vi "Read shortStatus.vi"(8 "error in (no error)":errorcluster, 11 "DomeController in":refnum<class "DomeController.lvclass">) -> (0 "error out":errorcluster, 2 "shortStatus":T1 {"azimuthAngle" min=0.0 max=360.0; "openingPercentage" min=0.0 max=100.0; "mainDoorOpeningPercentage" min=0.0 max=100.0}, 3 "DomeController out":refnum<class "DomeController.lvclass">)   [LabVIEW 2016, in "DomeController.lvclass"]
uses:
  DomeController.lvclass
  domeCommunicator/ComTypedefs/shortStatus.ctl
  domeCommunicator/ComTypedefs/openingStates.ctl
  IDome/domeTypedefs/openingPercentage.ctl
  domeCommunicator/ComTypedefs/sensorCode.ctl
  domeCommunicator/ComTypedefs/azimimuthPositionStatus.ctl
  IDome/domeTypedefs/azimuth.ctl
  IDome/domeTypedefs/direction.ctl
  IDome/domeTypedefs/domeState.ctl
  IDome/domeTypedefs/motionDirection.ctl
  IDome/domeTypedefs/openingMotion.ctl
  DomeController.lvclass/DomeController.ctl
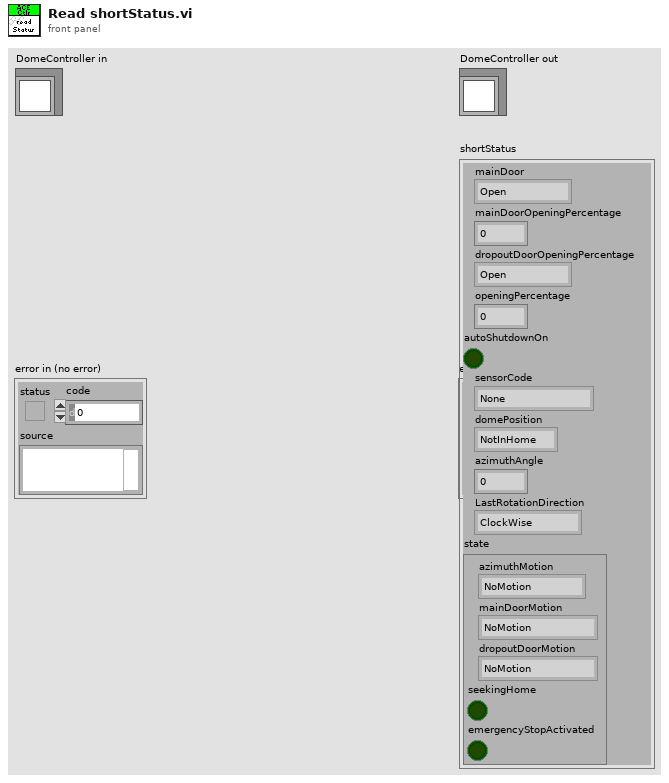
[diagram p1: front panel]
types:
  T1 = typedef "shortStatus.ctl" = cluster{"mainDoor":T2, "mainDoorOpeningPercentage":T3, "dropoutDoorOpeningPercentage":T2, "openingPercentage":T3, "autoShutdownOn":bool, "sensorCode":T4, "domePosition":T5, "azimuthAngle":T6, "LastRotationDirection":T7, "state":T8}
  T2 = typedef "openingStates.ctl" = enum16{"Open", "Shut", "Ajar"}
  T3 = typedef "openingPercentage.ctl" = dbl
  T4 = typedef "sensorCode.ctl" = enum16{"None", "RainSnowSensorTriggered", "CloudSensorTriggered", "BothSensorsTriggered"}
  T5 = typedef "azimimuthPositionStatus.ctl" = enum16{"NotInHome", "Home"}
  T6 = typedef "azimuth.ctl" = dbl
  T7 = typedef "direction.ctl" = enum16{"ClockWise", "CounterClockWise"}
  T8 = typedef "domeState.ctl" = cluster{"azimuthMotion":T9, "mainDoorMotion":T10, "dropoutDoorMotion ":T10, "seekingHome":bool, "emergencyStopActivated":bool}
  T9 = typedef "motionDirection.ctl" = enum16{"NoMotion", "MovingClockWise", "MovingCounterClockWise"}
  T10 = typedef "openingMotion.ctl" = enum16{"NoMotion", "Opening", "Closing"}
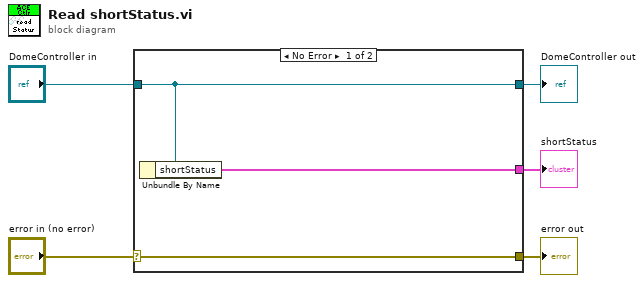
[diagram p0: block diagram]
diagram:
  n1 = case shown="No Error" "error in (no error)" {
    selector: "error in (no error)" -> [w8 w9]
    tunnel: [w8 w9] -> w4
    tunnel: [w7 w10] -> w2
    tunnel: "DomeController in" -> [w7 w10]
    tunnel: [w6 _] -> w1
    frame No Error {
      n2 = Unbundle By Name(w7) -> ("shortStatus"=w6:T1)
    }
    frame Error {
    }
  }
  "error out" <- w4
  "DomeController out" <- w2
  "shortStatus" <- w1
